vi "Init Queue.vi"(8 "error in":errorcluster) -> (0 "error out":errorcluster, 3 "Queue out":refnum<queue>)   [LabVIEW 2016]
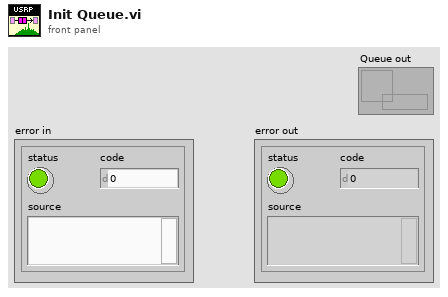
[diagram p1: front panel]
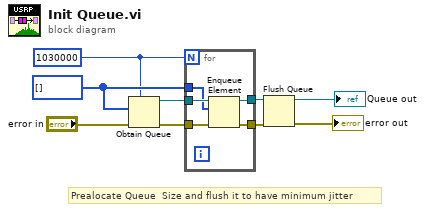
[diagram p0: block diagram]
diagram:
  w4 = 1030000
  w9 = u64[] [] ("subarray")
  # "Prealocate Queue  Size and flush it to have minimum jitter"
  n1 = Obtain Queue(max queue size (-1, unlimited)=w4, element data type=w9, error in (no error)="error in") -> (queue out=w2:refnum<queue>, error out=w3:errorcluster)  [unwired: 2 in, 1 out]
  n2 = for {
    N: w4 -> [_]
    tunnel: w2 -> [w14]
    tunnel: w3 -> [w13]
    tunnel: [w12] -> w6
    tunnel: [w11] -> w5
    tunnel: w9 -> [w10]
    n3 = Enqueue Element(queue=w14, element=w10, error in (no error)=w13) -> (queue out=w12:refnum<queue>, error out=w11:errorcluster)  [unwired: 1 in, 1 out]
  }
  n4 = Flush Queue(queue=w6, error in (no error)=w5) -> (queue out=→"Queue out":refnum<queue>, error out=→"error out":errorcluster)  [unwired: 1 out]
